vi "LogEngine.LogFile.Convert.vi"(8 "error in (no error)":errorcluster, 11 "path":path) -> (0 "error out":errorcluster, 2 "Status":string)   [LabVIEW 2025, in "XNET Bus Monitor Client.lvlib"]
uses:
  XNET Bus Monitor Client.lvlib
  bus_monitor_client/RPC Messages/ni_bus_monitor_api_Frame.ctl
  <vilib>/dlg_ctls.llb/Space Constant.vi
  <vilib>/Utility/error.llb/Trim Whitespace.vi
  Convert.TimeToUTCString.vi
  <vilib>/Utility/error.llb/Trim Whitespace One-Sided.vi
  bus_monitor_client/bus_monitor_client.lvlib
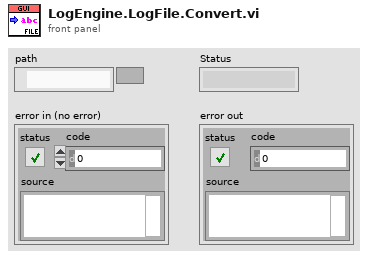
[diagram p1: front panel]
types:
  T1 = typedef "bus_monitor_client.lvlib/ni_bus_monitor_api_Frame.ctl" = cluster{"timestamp":dbl, "payload":u8[], "identifier":u32, "frame_type":u32, "extended":bool, "echo":bool}
  T2 = enum16{"open", "replace", "create", "open or create", "replace or create", "replace or create with confirmation"}
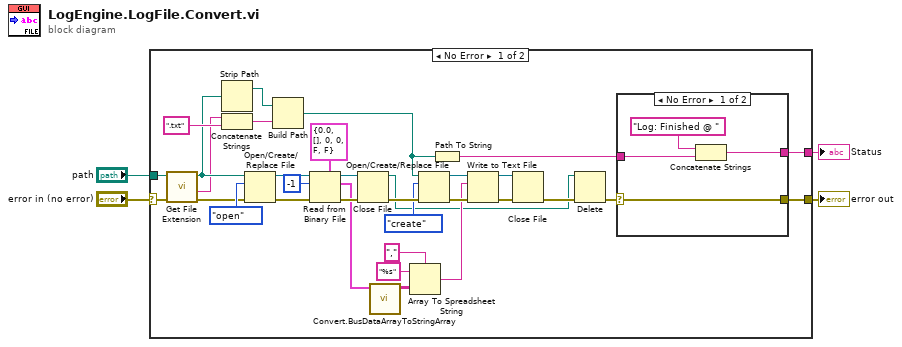
[diagram p0: block diagram]
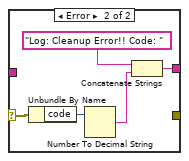
[diagram p2: hidden frame]
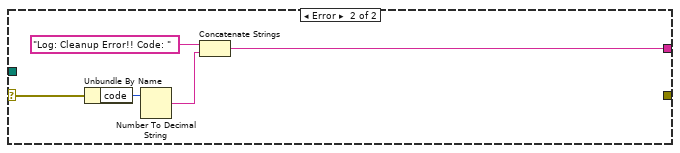
[diagram p3: hidden frame]
diagram:
  n1 = case shown="No Error" "error in (no error)" {
    selector: "error in (no error)" -> [w20 w49]
    tunnel: "path" -> [w26 _]
    tunnel: [w17 _] -> w2
    tunnel: [w18 w47] -> w4
    frame No Error {
      n2 = call <vilib>:"Get File Extension.vi"("error in (no error)"=w20, "file"=w26) -> ("error out"=w21:errorcluster, "filename without extension"=w19:string, "dup file"=w22:path)  [unwired: 5 in, 2 out]
      n3 = Strip Path(path=w22) -> (stripped path=w8:path)  [unwired: 1 out]
      n4 = Concatenate Strings(w19, ".txt" ("string")) -> (w24:string)
      n5 = Open/Create/Replace File(file path (use dialog)=w22, error in=w21, operation (0:open)=T2."open") -> (refnum out=w35:refnum<file>, error out=w36:errorcluster)  [unwired: 3 in, 1 out]
      n6 = Build Path(base path=w8, name or relative path=w24) -> (appended path=w6:path)
      n7 = Read from Binary File(5:T1 {"timestamp"=0.0, "payload"=[], "identifier"=0, "frame_type"=0, "extended"=FALSE, "echo"=FALSE} ("ni_xnet_can_bm_api_Frame"), 8:w36, 10:-1 ("count (1)"), 11:w35) -> (0:w29:errorcluster, 2:w12:T1[], 3:w27:refnum<file>)  [unwired: 2 in, 1 out]
      n8 = Close File(refnum=w27, error in=w29) -> (path=w9:path, error out=w28:errorcluster)
      n9 = call "Convert.BusDataArrayToStringArray.vi"("frame"=w12) -> ("Array out"=w16:string[][])  [unwired: 10 in]
      n10 = Array To Spreadsheet String(delimiter (Tab)=",", array=w16, 3:"%s" ("format string")) -> (spreadsheet string=w13:string)
      n11 = Open/Create/Replace File(file path (use dialog)=w6, error in=w28, operation (0:open)=T2."create") -> (refnum out=w33:refnum<file>, error out=w32:errorcluster)  [unwired: 3 in, 1 out]
      n12 = Path To String(path=w6) -> (string=w5:string)
      n13 = Write to Text File(file (use dialog)=w33, text=w13, error in=w32) -> (refnum out=w31:refnum<file>, error out=w30:errorcluster)  [unwired: 1 in, 1 out]
      n14 = Close File(refnum=w31, error in=w30) -> (error out=w11:errorcluster)  [unwired: 1 out]
      n15 = Delete(path (use dialog)=w9, error in=w11) -> (error out=w10:errorcluster)  [unwired: 3 in, 2 out]
      n16 = case shown="No Error" w10 {
        selector: w10 -> [w39 w43]
        tunnel: [w40 w42] -> w18
        tunnel: [w39 _] -> w17
        tunnel: w5 -> [w38 _]
        frame No Error {
          n17 = Concatenate Strings("Log: Finished @ " ("string"), w38) -> (w40:string)
        }
        frame Error {
          n18 = Unbundle By Name(w43) -> ("code"=w45:i32)
          n19 = Number To Decimal String(number=w45) -> (decimal integer string=w46:string)  [unwired: 1 in]
          n20 = Concatenate Strings("Log: Cleanup Error!! Code: ", w46) -> (w42:string)
        }
      }
    }
    frame Error {
      n21 = Unbundle By Name(w49) -> ("code"=w51:i32)
      n22 = Number To Decimal String(number=w51) -> (decimal integer string=w50:string)  [unwired: 1 in]
      n23 = Concatenate Strings("Log: Cleanup Error!! Code: ", w50) -> (w47:string)
    }
  }
  "Status" <- w4
  "error out" <- w2
